vi "goToHome.vi"(0 "Pmx4exSaController in":refnum<class "Pmx4exSaController.lvclass">, 1 "axis":T2, 2 "dir":T1, 3 "mode":T3, 5 "error in (no error)":errorcluster) -> (14 "Pmx4exSaController out":refnum<class "Pmx4exSaController.lvclass">, 17 "success?":bool, 18 "response":string, 19 "error out":errorcluster)   [LabVIEW 2013, in "classes.lvlib" / "Pmx4exSaController.lvclass"]
doc: "Produced By:\n\n<B>Kod Integrations, LLC</B>\n4835 Marianne Drive\nMount Airy, MD 21771\nhttp://www.kodintegrations.com\nemail: info@kodintegrations.com\nphone: (240) 687-1288"
uses:
  Pmx4exSaController.lvclass
  homing_mode.ctl
  axis.ctl
  linear_direction.ctl
  _Controller.lvclass
  common.lvlib
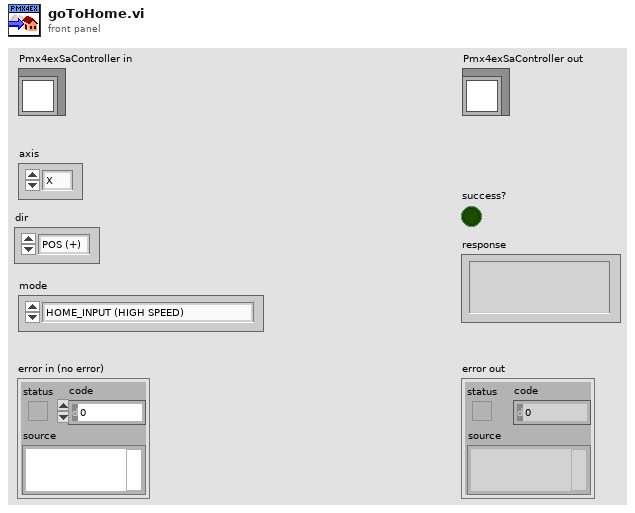
[diagram p1: front panel]
types:
  T1 = typedef "common.lvlib/linear_direction.ctl" = enum16{"POS (+)", "NEG (-)"}
  T2 = typedef "common.lvlib/axis.ctl" = enum16{"X", "Y", "Z", "U"}
  T3 = typedef "common.lvlib/homing_mode.ctl" = enum16{"HOME_INPUT (HIGH SPEED)", "LIMIT_INPUT", "HOME_INPUT_&_Z-INDEX", "Z-INDEX", "HOME_INPUT (HIGH_&_LOW_SPEED)"}
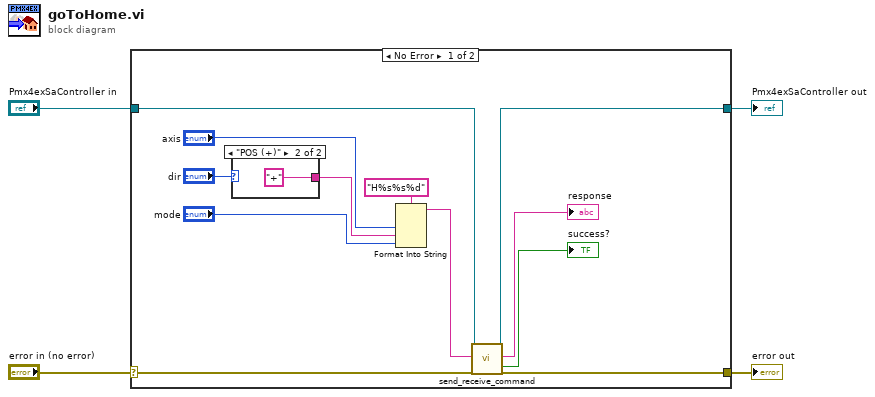
[diagram p0: block diagram]
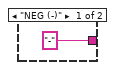
[diagram p2: hidden frame]
diagram:
  n1 = case shown="No Error" "error in (no error)" {
    selector: "error in (no error)" -> [w11 w20]
    tunnel: [w10 w20] -> w3
    tunnel: [w7 w19] -> w1
    tunnel: "Pmx4exSaController in" -> [w8 w19]
    frame No Error {
      n2 = case shown="\"POS (+)\"" "dir" {
        tunnel: ["-" "+"] -> w15
        frame "NEG (-)" {
        }
        frame "POS (+)" {
        }
      }
      n3 = Format Into String(format string="H%s%s%d", "axis", w15, "mode") -> (resulting string=w9:string)  [unwired: 2 in, 1 out]
      n4 = call "send_receive_command.vi"("reference (in)"=w8, "ASCII Command (in)"=w9, "error in (no error)"=w11) -> ("reference (out)"=w7:refnum<class "Pmx4exSaController.lvclass">, "response (out)"=→"response":string, "success?"=→"success?":bool, "error out"=w10:errorcluster)  [unwired: 12 in, 1 out]
    }
    frame Error {
    }
  }
  "error out" <- w3
  "Pmx4exSaController out" <- w1
